vi "Bool parse tests.vi"() -> ()   [LabVIEW 2015]
uses:
  API/JSON Document Class/json parse/poly instances/json Parse Boolean - string path.vi
  API/JSON Document Class/json parse/poly instances/json Parse Boolean Array - string path.vi
  API/JSON Document Class/JSON Document.lvclass
panel:
  out "elements defaulted?":bool[](array[boolean])
  out "value 3":bool[](array[boolean])
  out "defaulted? 3":bool
  out "defaulted? 2":bool
  out "value 2":bool
  out "value":bool
  out "defaulted?":bool
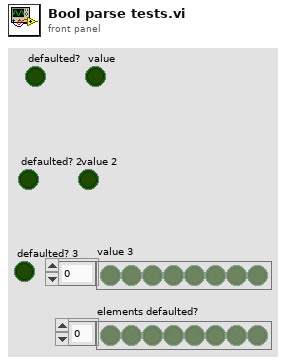
[diagram p1: front panel]
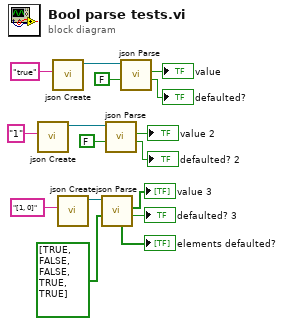
[diagram p0: block diagram]
diagram:
  n1 = call "json Create.vi"("JSON String"="1") -> ("JSON Document out"=w8:refnum<class "JSON Document.lvclass">)  [unwired: 9 in, 1 out]
  n2 = call "json Create.vi"("JSON String"="true") -> ("JSON Document out"=w15:refnum<class "JSON Document.lvclass">)  [unwired: 9 in, 1 out]
  n3 = call "json Create.vi"("JSON String"="[1, 0]") -> ("JSON Document out"=w5:refnum<class "JSON Document.lvclass">)  [unwired: 9 in, 1 out]
  n4 = call-poly "json Parse.vi"("default"=bool[] [TRUE, FALSE, FALSE, TRUE, TRUE], "JSON Document in"=w5) -> ("defaulted?"=→"defaulted? 3":bool, "value"=→"value 3":bool[], "elements defaulted?"=→"elements defaulted?":bool[])  [unwired: 5 in, 2 out]
  n5 = call-poly "json Parse.vi"("default"=FALSE, "JSON Document in"=w8) -> ("defaulted?"=→"defaulted? 2":bool, "value"=→"value 2":bool)  [unwired: 6 in, 2 out]
  n6 = call-poly "json Parse.vi"("default"=FALSE, "JSON Document in"=w15) -> ("defaulted?"=→"defaulted?":bool, "value"=→"value":bool)  [unwired: 6 in, 2 out]
